vi "Test Process Multiple Start Does Not Change State of Process.vi"(8 "error in (no error)":errorcluster, 11 "Process Test In":refnum<class "Process Test.lvclass">) -> (0 "error out":errorcluster, 3 "Process Test Out":refnum<class "Process Test.lvclass">)   [LabVIEW 2020, in "Process Test.lvclass"]
uses:
  Process Test.lvclass
  C:/Program Files (x86)/National Instruments/LabVIEW 2020/vi.lib/Asteme/LUnit/Test Case.lvclass
  Framework/Process/Process.lvclass/Process.ctl
  <vilib>/Asteme/LUnit/Test Case.lvclass/Test Case.ctl
  <vilib>/Asteme/LUnit/LUnit Assertion Result.lvclass/LUnit Assertion Result.ctl
  Framework/Process/Public/Get Lifecycle State.vi
  Framework/Process/Private/SubVIs/Wait for finish.vi
  Framework/Process/Protected/Messaging/Enqueue Message.vi
  Framework/Process/Private/SubVIs/Set Lifecycle State.vi
  <vilib>/Asteme/LUnit/Palette/Fail.vi
  <vilib>/Asteme/LUnit/Palette/Pass.vi
  <vilib>/Asteme/LUnit/Set Assertion Type.vi
  <vilib>/Utility/error.llb/Clear Errors.vi
  <vilib>/Asteme/LUnit/Add test result.vi
  <vilib>/Asteme/LUnit/LUnit Write Passed.vi
  <vilib>/Asteme/LUnit/LUnit Get Test Case.vi
  <vilib>/Asteme/LUnit/LUnit Write Message.vi
  <vilib>/Asteme/LUnit/LUnit Write Description.vi
  <vilib>/Asteme/LUnit/LUnit Write Assertion Type.vi
  <vilib>/Asteme/LUnit/Read Test Case Name.vi
  <vilib>/Utility/error.llb/Error Cluster From Error Code.vi
  <vilib>/Asteme/LUnit/Assertion Result/LUnit Get Test Name.vi
  <vilib>/Asteme/LUnit/LUnit Assertion Result.lvclass
  Framework/Process/Process.lvclass
  <vilib>/Asteme/LUnit/Test Case.lvclass
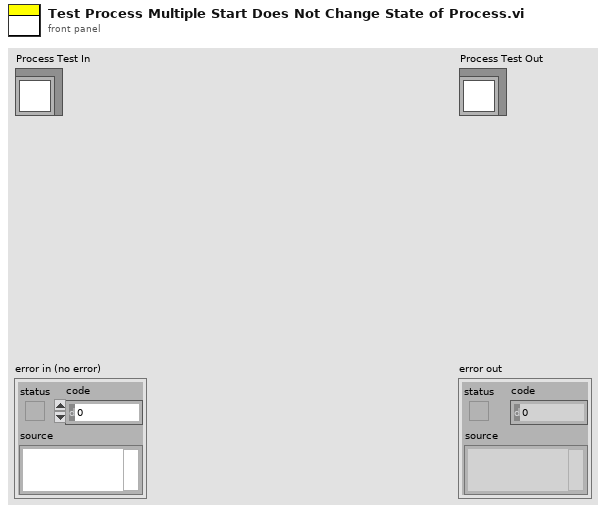
[diagram p1: front panel]
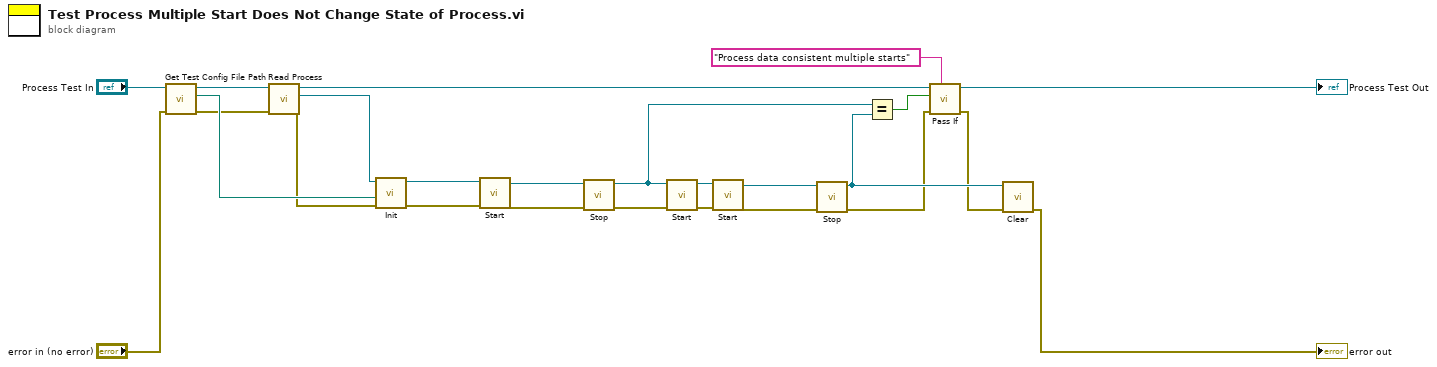
[diagram p0: block diagram]
diagram:
  n1 = call-dynamic "Get Test Config File Path.vi"("error in (no error)"="error in (no error)", "Base Class Test in"="Process Test In") -> ("error out"=w14:errorcluster, "Test config path"=w18:path, "Base Class Test out"=w20:refnum<class "Process Test.lvclass">)  [unwired: 7 in]
  n2 = call "Read Process.vi"("error in (no error)"=w14, "Process Test in"=w20) -> ("error out"=w15:errorcluster, "Process.lvclass"=w16:refnum<class "Process.lvclass">, "Process Test out"=w17:refnum<class "Process Test.lvclass">)  [unwired: 7 in]
  n3 = call-dynamic "Init.vi"("error in (no error)"=w15, "Config File Path"=w18, "Process In"=w16) -> ("error out"=w21:errorcluster, "Process Out"=w22:refnum<class "Process.lvclass">)  [unwired: 7 in]
  n4 = call "Start.vi"("error in (no error)"=w21, "Process In"=w22) -> ("error out"=w24:errorcluster, "Process Out"=w25:refnum<class "Process.lvclass">)  [unwired: 8 in]
  n5 = call "Stop.vi"("error in (no error)"=w24, "Process In"=w25) -> ("error out"=w2:errorcluster, "Process Out"=w10:refnum<class "Process.lvclass">)  [unwired: 7 in, 1 out]
  n6 = call "Start.vi"("error in (no error)"=w2, "Process In"=w10) -> ("error out"=w1:errorcluster, "Process Out"=w3:refnum<class "Process.lvclass">)  [unwired: 8 in]
  n7 = call "Start.vi"("error in (no error)"=w1, "Process In"=w3) -> ("error out"=w12:errorcluster, "Process Out"=w11:refnum<class "Process.lvclass">)  [unwired: 8 in]
  n8 = call "Stop.vi"("error in (no error)"=w12, "Process In"=w11) -> ("error out"=w6:errorcluster, "Process Out"=w9:refnum<class "Process.lvclass">)  [unwired: 7 in, 1 out]
  n9 = Equal?(x=w10, y=w9) -> (x = y?=w7:bool)
  n10 = call <vilib>:"Pass If.vi"("Description"="Process data consistent multiple starts", "error in (no error)"=w6, "Pass?"=w7, "Test Case In"=w17) -> ("error out"=w5:errorcluster, "Test Case Out"=→"Process Test Out":refnum<class "Process Test.lvclass">)  [unwired: 6 in]
  n11 = call-dynamic "Clear.vi"("error in (no error)"=w5, "Process In"=w9) -> ("error out"=→"error out":errorcluster)  [unwired: 8 in, 1 out]
